vi "time_frame(SubVI).vi"(8 "error in (no error)":errorcluster, 11 "Application in":refnum<vi>) -> (0 "error out":errorcluster, 2 "Numeric":sgl, 3 "Application out":refnum<vi>)   [LabVIEW 2014]
uses:
  <userlib>/Nanonis Prog Interface V5/Nanonis Prog Interface.lvlib
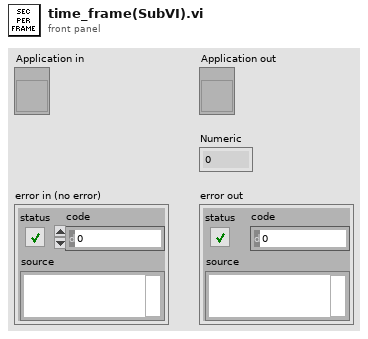
[diagram p1: front panel]
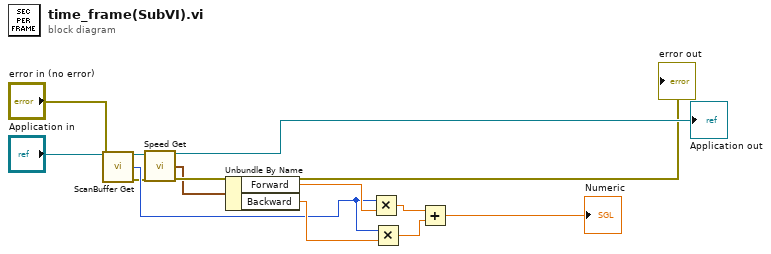
[diagram p0: block diagram]
diagram:
  n1 = call <userlib>:"ScanBuffer Get.vi"("Application ref in"="Application in", "error in (no error)"="error in (no error)") -> ("Application ref out"=w1:refnum<vi>, "Pixels/line"=w4:i32, "error out"=w2:errorcluster)  [unwired: 9 in, 2 out]
  n2 = call <userlib>:"Speed Get.vi"("Application ref in"=w1, "error in (no error)"=w2) -> ("Application ref out"=→"Application out":refnum<vi>, "Time/line (s)"=w3:cluster{"Forward":sgl, "Backward":sgl}, "error out"=→"error out":errorcluster)  [unwired: 8 in, 3 out]
  n3 = Unbundle By Name(w3) -> ("Forward"=w5:sgl, "Backward"=w6:sgl)
  n4 = Multiply(x=w4, y=w5) -> (x*y=w8:sgl)
  n5 = Multiply(x=w4, y=w6) -> (x*y=w7:sgl)
  n6 = Add(x=w8, y=w7) -> (x+y=→"Numeric":sgl)
